vi "test Flatten Unflatten 1.1.vi"(8 "error in (no error)":errorcluster, 11 "TestCase in":refnum<class "Configuration Tests.lvclass">) -> (0 "error out":errorcluster, 3 "TestCase out":refnum<class "Configuration Tests.lvclass">)   [LabVIEW 2017, in "Configuration Tests.lvclass"]
uses:
  Configuration Tests.lvclass
  Typedefs/DSF Version Info.ctl
  Configuration Tests.lvclass/Configuration Tests.ctl
  Classes/Configuration/Configuration Session.lvclass
  DSF Core.lvlib
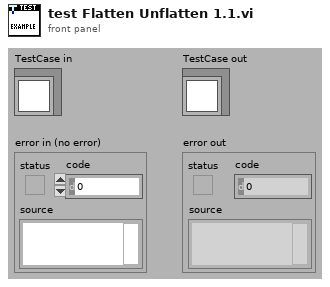
[diagram p1: front panel]
types:
  T1 = typedef "DSF Core.lvlib/DSF Version Info.ctl" = cluster{"major":u32, "minor":u32, "fix":u32, "build":string}
  T2 = typedef "DSF Core.lvlib/DSF Engine Framework Configuration.ctl" = cluster{"plugins":T3[]}
  T3 = typedef "DSF Core.lvlib/DSF Engine Plugin Configuration.ctl" = cluster{"name":string, "components":string[], "cycle timing":T4, "threads":T5[], "transfer groups":T7[], "settings":T6}
  T4 = typedef "DSF Core.lvlib/DSF Timing Info.ctl" = cluster{"priority":u64, "decimation":u64, "offset":u64}
  T5 = typedef "DSF Core.lvlib/DSF Engine Plugin Thread Configuration.ctl" = cluster{"buffer converter settings":T6, "transceiver settings":T6, "custom settings":T6, "processor":i32, "priority offset":i16}
  T6 = typedef "DSF Core.lvlib/DSF Settings Info.ctl" = cluster{"key":string, "value":string}[]
  T7 = typedef "DSF Core.lvlib/DSF Engine Transfer Group Configuration.ctl" = cluster{"name":string, "direction":T8, "cycle timing":T4, "thread index":i32, "settings":T6, "transfers":T9[], "timeout behavior":T13}
  T8 = typedef "DSF Core.lvlib/DSF Direction.ctl" = enum8{"Tx", "Rx"}
  T9 = typedef "DSF Core.lvlib/DSF Engine Transfer Configuration.ctl" = cluster{"name":string, "byte order":T10, "settings":T6, "channels":T11[]}
  T10 = typedef "DSF Core.lvlib/DSF Byte Order.ctl" = enum8{"big-endian", "little-endian"}
  T11 = typedef "DSF Core.lvlib/DSF Engine Channel Configuration.ctl" = cluster{"string offset":u64, "string data type":T12, "engine data type":T12, "name":string, "settings":T6, "units":string}
  T12 = typedef "DSF Core.lvlib/DSF Data Type.ctl" = enum8{"Bool", "SGL", "DBL", "I8", "I16", "I32", "I64", "U8", "U16", "U32", "U64"}
  T13 = typedef "DSF Core.lvlib/DSF Timeout Behavior.ctl" = enum8{"Increment Late Count", "Throw Error"}
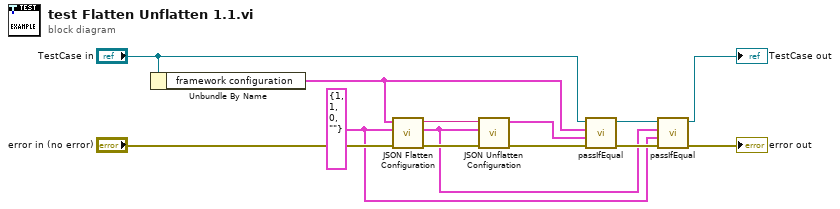
[diagram p0: block diagram]
diagram:
  w4 = T1 {"major"=1, "minor"=1, "fix"=0, "build"=""} ("dsf version")
  n1 = Unbundle By Name("TestCase in") -> ("framework configuration"=w1:T2)
  n2 = call "JSON Flatten Configuration.vi"("error in (no error)"="error in (no error)", "dsf version"=w4, "framework configuration"=w1) -> ("error out"=w12:errorcluster, "actual dsf version"=w3:T1, "dsf configuration json"=w11:string)  [unwired: 6 in]
  n3 = call "JSON Unflatten Configuration.vi"("error in (no error)"=w12, "dsf version"=w3, "dsf configuration json"=w11) -> ("error out"=w9:errorcluster, "framework configuration"=w10:T2)  [unwired: 7 in]
  n4 = call-dynamic "passIfEqual.vi"("error in (no error)"=w9, "y"=w10, "x"=w1, "TestCase in"="TestCase in") -> ("error out"=w8:errorcluster, "TestCase out"=w7:refnum<class "Configuration Tests.lvclass">)  [unwired: 6 in]
  n5 = call-dynamic "passIfEqual.vi"("error in (no error)"=w8, "y"=w4, "x"=w3, "TestCase in"=w7) -> ("error out"=→"error out":errorcluster, "TestCase out"=→"TestCase out":refnum<class "Configuration Tests.lvclass">)  [unwired: 6 in]
